vi "Prep_Logfile_And_Save_Paths.vi"(0 "Data Directory":path, 1 "Session Name":string, 2 "upper":dbl caption="Upper Cut-Off", 3 "lower":dbl caption="Lower Cut-Off", 4 "MVC Number":dbl, 5 "rate":dbl caption="Upper Cut-Off", 6 "MVC Duration (s)":dbl, 7 "fps":dbl caption="Lower Cut-Off", 8 "EMG Channel To Display":dbl, 9 "dispSize":dbl caption="Lower Cut-Off", 11 "mvcSize":dbl caption="Upper Cut-Off") -> (14 "log filepath":path, 15 "MVC Raw Path":path, 16 "MVC Filtered Path":path, 18 "GetMaxStartTime":timestamp, 19 "error out":errorcluster)   [LabVIEW 2016]
uses:
  <vilib>/Utility/file.llb/Write Delimited Spreadsheet (string).vi
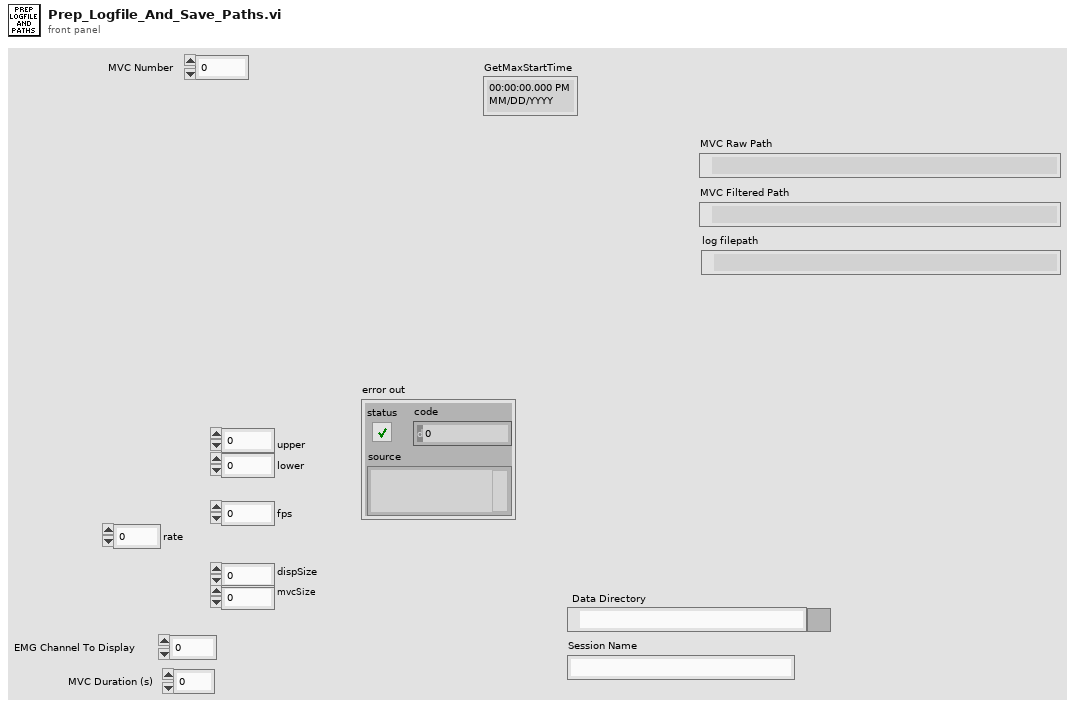
[diagram p1: front panel]
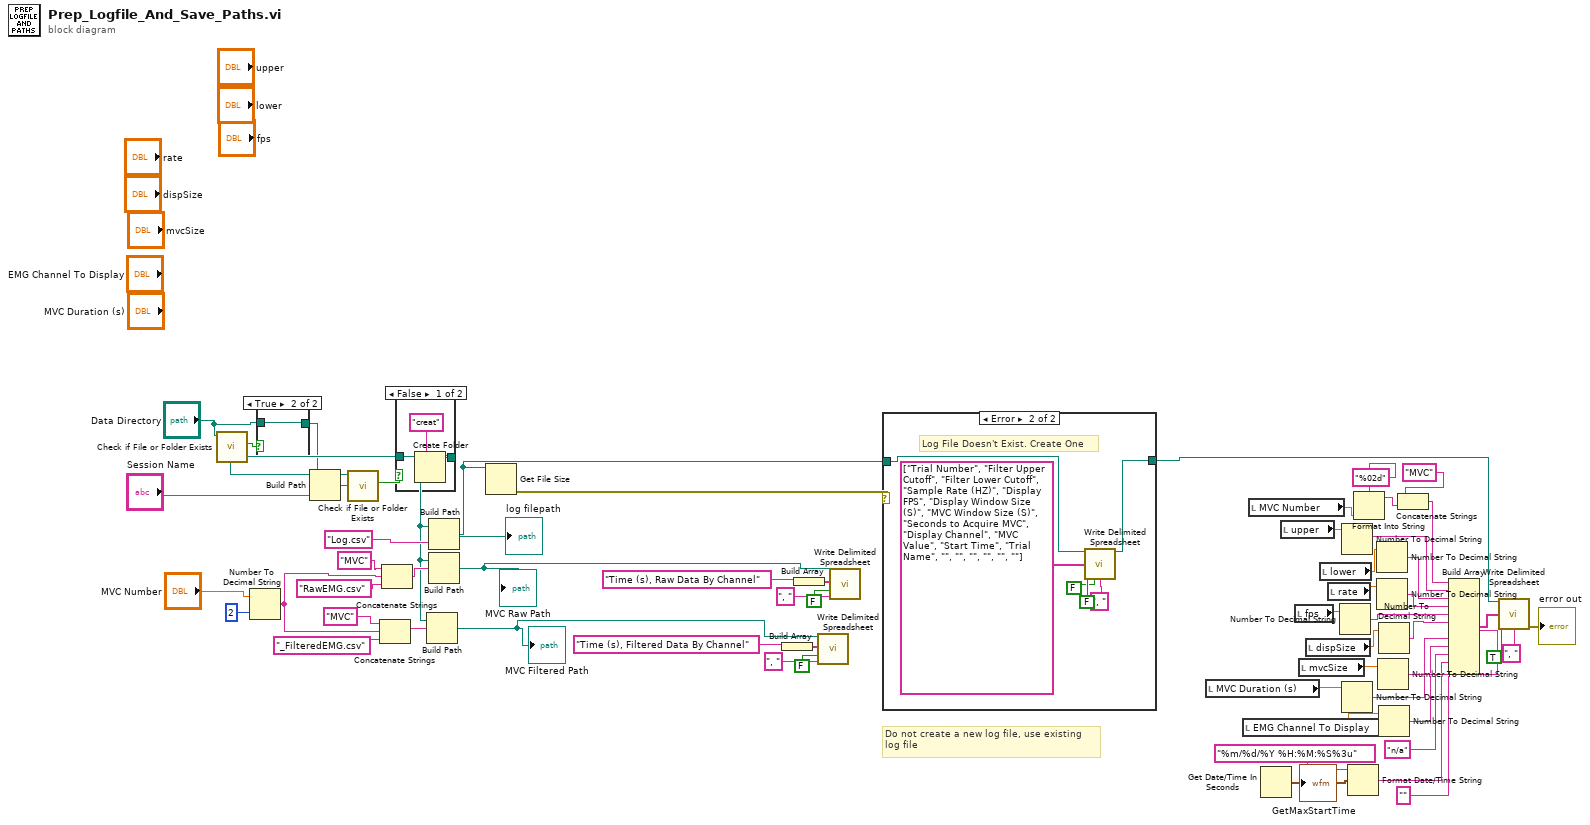
[diagram p0: block diagram]
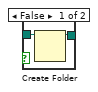
[diagram p4: hidden frame]
diagram:
  # "Do not create a new log file, use existing \nlog file"
  n1 = call <vilib>:"Check if File or Folder Exists.vi"("path"="Data Directory") -> ("file or folder exists?"=w17:bool)  [unwired: 8 in, 2 out]
  n2 = Number To Decimal String(number="MVC Number", width (-)=i16 2) -> (decimal integer string=w38:string)
  n3 = case shown="True" w17 {
    tunnel: [w63 w64] -> w52
    tunnel: "Data Directory" -> [w62 w64]
    frame False {
      n4 = Create Folder(path (use dialog)=w62) -> (created path=w63:path)  [unwired: 2 in, 2 out]
    }
    frame True {
    }
  }
  n5 = Build Path(base path=w52, name or relative path="Session Name") -> (appended path=w55:path)
  n6 = call <vilib>:"Check if File or Folder Exists.vi"("path"=w55) -> ("file or folder exists?"=w54:bool, "dup path"=w53:path)  [unwired: 8 in, 1 out]
  n7 = Concatenate Strings("MVC" ("string"), w38, "_FilteredEMG.csv" ("string")) -> (w60:string)
  n8 = Concatenate Strings("MVC" ("string"), w38, "RawEMG.csv" ("string")) -> (w59:string)
  n9 = case shown="False" w54 {
    tunnel: w53 -> [w67 w68]
    tunnel: [w66 w68] -> w49
    frame False {
      n10 = Create Folder(prompt (Create Folder)="creat", path (use dialog)=w67) -> (created path=w66:path)  [unwired: 1 in, 2 out]
    }
    frame True {
    }
  }
  n11 = Build Path(base path=w49, name or relative path=w60) -> (appended path=w1:path)
  "MVC Filtered Path" <- w1
  n12 = Build Path(base path=w49, name or relative path="Log.csv" ("string")) -> (appended path=w13:path)
  "log filepath" <- w13
  n13 = Build Path(base path=w49, name or relative path=w59) -> (appended path=w6:path)
  "MVC Raw Path" <- w6
  n14 = Get File Size(file=w13) -> (0:w15:errorcluster)  [unwired: 1 in, 2 out]
  n15 = Build Array("Time (s), Filtered Data By Channel" ("time format string (%c)")) -> (w3:string[])
  n16 = Build Array("Time (s), Raw Data By Channel" ("time format string (%c)")) -> (w8:string[])
  n17 = call-poly <vilib>:"Write Delimited Spreadsheet.vi"("file path (dialog if empty)"=w1, "1D data"=w3, "append to file? (new file:F)"=FALSE, "delimiter (\\t)"=", " ("delimiter (\\t)")) -> ()  [unwired: 10 in, 2 out]
  n18 = call-poly <vilib>:"Write Delimited Spreadsheet.vi"("file path (dialog if empty)"=w6, "1D data"=w8, "append to file? (new file:F)"=FALSE, "delimiter (\\t)"=", " ("delimiter (\\t)")) -> ()  [unwired: 10 in, 2 out]
  n19 = case shown="Error" w15 {
    tunnel: [w69 w71] -> w29
    tunnel: w13 -> [w69 w70]
    frame No Error {
    }
    frame Error {
      # "Log File Doesn't Exist. Create One"
      n20 = call-poly <vilib>:"Write Delimited Spreadsheet.vi"("file path (dialog if empty)"=w70, "1D data"=string[] ["Trial Number", "Filter Upper Cutoff", "Filter Lower Cutoff", "Sample Rate (HZ)", "Display FPS", "Display Window Size (S)", "MVC Window Size (S)", "Seconds to Acquire MVC", "Display Channel", "MVC Value", "Start Time", "Trial Name", "", "", "", "", "", ""], "append to file? (new file:F)"=FALSE, "transpose? (no:F)"=FALSE, "delimiter (\\t)"=", " ("delimiter (\\t)")) -> ("new file path (Not A Path if cancelled)"=w71:path)  [unwired: 9 in, 1 out]
    }
  }
  n21 = local read "MVC Duration (s)"() -> (w43:dbl)
  n22 = local read "EMG Channel To Display"() -> (w42:dbl)
  n23 = local read "MVC Number"() -> (w25:dbl)
  n24 = Get Date/Time In Seconds() -> (seconds since 1Jan1904=w21:timestamp)
  "GetMaxStartTime" <- w21
  n25 = local read "upper"() -> (w48:dbl)
  n26 = local read "fps"() -> (w45:dbl)
  n27 = local read "mvcSize"() -> (w44:dbl)
  n28 = local read "dispSize"() -> (w39:dbl)
  n29 = local read "lower"() -> (w47:dbl)
  n30 = local read "rate"() -> (w46:dbl)
  n31 = Number To Decimal String(number=w45) -> (decimal integer string=w35:string)  [unwired: 1 in]
  n32 = Number To Decimal String(number=w48) -> (decimal integer string=w23:string)  [unwired: 1 in]
  n33 = Number To Decimal String(number=w43) -> (decimal integer string=w32:string)  [unwired: 1 in]
  n34 = Format Date/Time String(time format string (%c)="%m/%d/%Y %H:%M:%S%3u", seconds (now)=w21) -> (date/time string=w19:string)  [unwired: 1 in]
  n35 = Format Into String(format string="%02d", w25) -> (resulting string=w28:string)  [unwired: 2 in, 1 out]
  n36 = Number To Decimal String(number=w47) -> (decimal integer string=w37:string)  [unwired: 1 in]
  n37 = Number To Decimal String(number=w46) -> (decimal integer string=w36:string)  [unwired: 1 in]
  n38 = Number To Decimal String(number=w44) -> (decimal integer string=w33:string)  [unwired: 1 in]
  n39 = Number To Decimal String(number=w39) -> (decimal integer string=w34:string)  [unwired: 1 in]
  n40 = Number To Decimal String(number=w42) -> (decimal integer string=w31:string)  [unwired: 1 in]
  n41 = Concatenate Strings("MVC" ("string"), w28) -> (w24:string)
  n42 = Build Array(w24, w23, w37, w36, w35, w34, w33, w32, w31, "n/a", w19, "" ("element")) -> (w41:string[])
  n43 = call-poly <vilib>:"Write Delimited Spreadsheet.vi"("file path (dialog if empty)"=w29, "1D data"=w41, "append to file? (new file:F)"=TRUE, "delimiter (\\t)"=", " ("delimiter (\\t)")) -> ("error out"=→"error out":errorcluster)  [unwired: 10 in, 1 out]
